vi "Init.vi"(8 "error in (no error)":errorcluster, 9 "Menu Items":refnum<data-value>[](array[refnum]), 11 "Menu in":refnum<class "MGI_Menu.lvclass">) -> (0 "error out":errorcluster, 2 "MenuItemStatusChange":refnum<user-event>, 3 "Menu out":refnum<class "MGI_Menu.lvclass">)   [LabVIEW 2016, in "MGI_Menu.lvclass"]
doc: "Inistializes the menu. This vi will delete any menu's that are currently in place. This also creates the Menuitem Clicked event.\n\nDo not use this VI to rebuild the menu. There is a separate Rebuild Menu VI.\n\nAuthored by Derek E. Trepanier\nsupport@mooregoodideas.com\nwww.mooregoodideas.com\n\nCopyright (c) 2012, Moore Good Ideas, Inc.\n\nAll rights reserved.\n\nRedistribution and use in source and binary forms, with or without modification, are permitted provided that the following conditions are met:\n\n * Redistributions of source code must retain the above copyright notice, this list of conditions and the following disclaimer.\n * Redistributions in binary form must reproduce the above copyright notice, this list of conditions and the following disclaimer in the documentation and/or other materials provided with the distribution.\n * Neither the name of Moore Good Ideas, Inc. nor the names of its contributors may be used to endorse or promote products derived from this software without specific prior written permission.\n\nTHIS SOFTWARE IS PROVIDED BY THE COPYRIGHT HOLDERS AND CONTRIBUTORS \"AS IS\" AND ANY EXPRESS OR IMPLIED WARRANTIES, INCLUDING, BUT NOT LIMITED TO, THE IMPLIED WARRANTIES OF MERCHANTABILITY AND FITNESS FOR A PARTICULAR PURPOSE ARE DISCLAIMED. IN NO EVENT SHALL THE COPYRIGHT OWNER OR CONTRIBUTORS BE LIABLE FOR ANY DIRECT, INDIRECT, INCIDENTAL, SPECIAL, EXEMPLARY, OR CONSEQUENTIAL DAMAGES (INCLUDING, BUT NOT LIMITED TO, PROCUREMENT OF SUBSTITUTE GOODS OR SERVICES; LOSS OF USE, DATA, OR PROFITS; OR BUSINESS INTERRUPTION) HOWEVER CAUSED AND ON ANY THEORY OF LIABILITY, WHETHER IN CONTRACT, STRICT LIABILITY, OR TORT (INCLUDING NEGLIGENCE OR OTHERWISE) ARISING IN ANY WAY OUT OF THE USE OF THIS SOFTWARE, EVEN IF ADVISED OF THE POSSIBILITY OF SUCH DAMAGE."
uses:
  <userlib>/_MGI/Menu Building/MenuTypes/MGI_Menu.lvclass
  <userlib>/_MGI/Menu Building/MenuItem/MGI_MenuItem.lvclass
  <userlib>/_MGI/Menu Building/MenuItemStatusChange/MGI_MenuItemStatusChange.lvclass
  <userlib>/_MGI/Menu Building/MenuTypes/MGI_Menu.lvclass/MGI_Menu.ctl
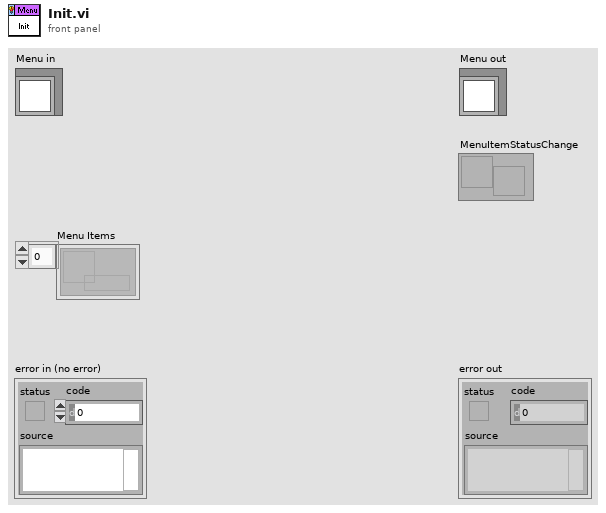
[diagram p1: front panel]
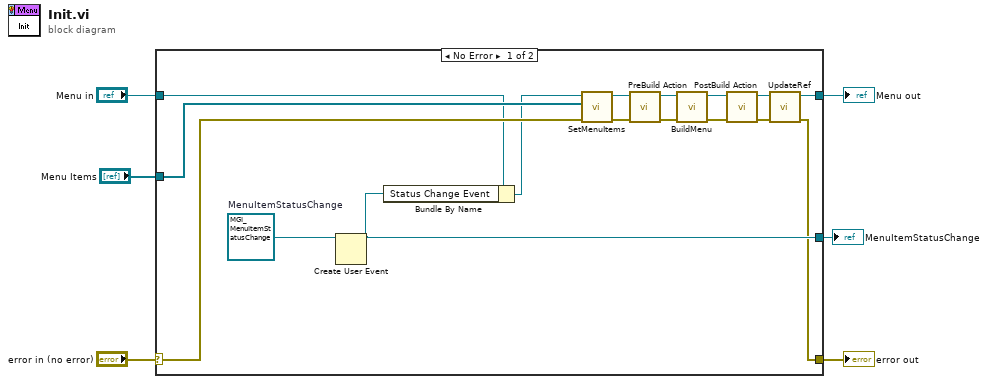
[diagram p0: block diagram]
diagram:
  n1 = case shown="No Error" "error in (no error)" {
    selector: "error in (no error)" -> [w16 w24]
    tunnel: [w7 w24] -> w5
    tunnel: [w9 w23] -> w3
    tunnel: "Menu in" -> [w12 w23]
    tunnel: "Menu Items" -> [w17 _]
    tunnel: [w18 _] -> w1
    frame No Error {
      w14 = refnum<class "MGI_MenuItemStatusChange.lvclass"> refnum  # MenuItemStatusChange
      n2 = Create User Event(user event datatype=w14) -> (user event=w18:refnum<user-event>)  [unwired: 1 in, 1 out]
      n3 = Bundle By Name(cluster=w12, "Status Change Event"=w18) -> (w11:refnum<class "MGI_Menu.lvclass">)
      n4 = call <userlib>:"SetMenuItems.vi"("error in (no error)"=w16, "Menu Items"=w17, "MGI_Menu in"=w11) -> ("error out"=w15:errorcluster, "MGI_Menu out"=w13:refnum<class "MGI_Menu.lvclass">)  [unwired: 7 in]
      n5 = call-dynamic "PreBuild Action.vi"("error in (no error)"=w15, "Menu in"=w13) -> ("error out"=w21:errorcluster, "Menu out"=w22:refnum<class "MGI_Menu.lvclass">)  [unwired: 8 in]
      n6 = call-dynamic "BuildMenu.vi"("error in (no error)"=w21, "Menu in"=w22) -> ("error out"=w19:errorcluster, "Menu out"=w20:refnum<class "MGI_Menu.lvclass">)  [unwired: 8 in]
      n7 = call-dynamic "PostBuild Action.vi"("error in (no error)"=w19, "Menu in"=w20) -> ("error out"=w8:errorcluster, "Menu out"=w10:refnum<class "MGI_Menu.lvclass">)  [unwired: 8 in]
      n8 = call <userlib>:"UpdateRef.vi"("error in (no error)"=w8, "Menu in"=w10) -> ("error out"=w7:errorcluster, "Menu out"=w9:refnum<class "MGI_Menu.lvclass">)  [unwired: 8 in]
    }
    frame Error {
    }
  }
  "error out" <- w5
  "Menu out" <- w3
  "MenuItemStatusChange" <- w1
